vi "Get LR700 R & X_GPIB.vi"(4 "error in (no error)":errorcluster, 7 "Instrument GPIB Addr.":i16=18) -> (0 "error out":errorcluster, 2 "X":dbl format="%.2e", 3 "Resistance":dbl format="%.4e")   [LabVIEW 2015]
uses:
  Get LR700 data_GPIB.vi
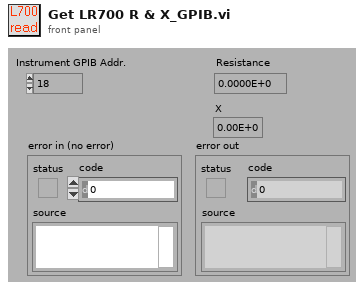
[diagram p1: front panel]
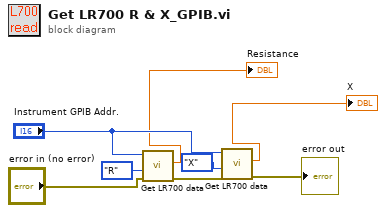
[diagram p0: block diagram]
diagram:
  n1 = call-poly "Get LR700 data.vi"("error in (no error)"="error in (no error)", "Data chanel"=enum16{"R", "X"}."R", "GPIB Addr"="Instrument GPIB Addr.") -> ("error out"=w6:errorcluster, "Data"=→"Resistance":dbl)  [unwired: 1 in, 2 out]
  n2 = call-poly "Get LR700 data.vi"("error in (no error)"=w6, "Data chanel"=enum16{"R", "X"}."X", "GPIB Addr"="Instrument GPIB Addr.") -> ("error out"=→"error out":errorcluster, "Data"=→"X":dbl)  [unwired: 1 in, 2 out]
